vi "Write.vi"(6 "Data":u8[](array[numeric]), 8 "Error In":errorcluster, 9 "Offset":i32 format="%.0x", 10 "Index Group":u32 format="%.0x", 11 "AMS Connection In":T1) -> (0 "Error Out":errorcluster, 1 "Success":bool, 2 "ADS Error":T3 items=["NoError"=0, "InternalError"=1, "NoRTime"=2, "LockedMemoryError"=3, "MailBoxError"=4, "WrongHMsg"=5, "TargetPortNotFound"=6, "TargetMachineNotFound"=7, "UnknownCommandID"=8, "BadTaskID"=9, "NoIO"=10, "UnknownAmsCommand"=11, "Win32Error"=12, "PortNotConnected"=13, "InvalidAmsLength"=14, "InvalidAmsNetID"=15, "AmsSyncAmsError"=22, "AmsSyncNoIndexMap"=23, "InvalidAmsPort"=24, "NoMemory"=25, "TCPSendError"=26, "HostUnreachable"=27, "NoLockedMemory"=1280, "MailboxFull"=1282, "DeviceError"=1792, "DeviceServiceNotSupported"=1793, "DeviceInvalidGroup"=1794, "DeviceInvalidOffset"=1795, "DeviceInvalidAccess"=1796, "DeviceInvalidSize"=1797, "DeviceInvalidData"=1798, "DeviceNotReady"=1799, "DeviceBusy"=1800, "DeviceInvalidContext"=1801, "DeviceNoMemory"=1802, "DeviceInvalidParam"=1803, "DeviceNotFound"=1804, "DeviceSyntaxError"=1805, "DeviceIncompatible"=1806, "DeviceExists"=1807, "DeviceSymbolNotFound"=1808, "DeviceSymbolVersionInvalid"=1809, "DeviceInvalidState"=1810, "DeviceTransModeNotSupported"=1811, "DeviceNotifyHandleInvalid"=1812, "DeviceClientUnknown"=1813, "DeviceNoMoreHandles"=1814, "DeviceInvalidWatchsize"=1815, "DeviceNotInitialized"=1816, "DeviceTimeOut"=1817, "DeviceNoInterface"=1818, "DeviceInvalidInterface"=1819, "DeviceInvalidCLSID"=1820, "DeviceInvalidObjectID"=1821, "ClientError"=1856, "ClientInvalidParameter"=1857, "ClientListEmpty"=1858, "ClientVariableInUse"=1859, "ClientDuplicateInvokeID"=1860, "ClientSyncTimeOut"=1861, "ClientW32OR"=1862, "ClientTimeoutInvalid"=1863, "ClientPortNotOpen"=1864, "ClientNoAmsAddr"=1865, "ClientSyncInternal"=1872, "ClientAddHash"=1873, "ClientRemoveHash"=1874, "ClientNoMoreSymbols"=1875, "ClientSyncResInvalid"=1876, "ClientSyncPortLocked"=1877, "ClientQueueFull"=1878], 3 "AMS Connection Out":T1)   [LabVIEW 2019, in "TwinCAT ADS.lvlib"]
uses:
  <userlib>/PMA/TwinCAT ADS.lvlib
  <userlib>/PMA/Low Level/TypeDefs/AMS Connection.ctl
  <userlib>/PMA/Low Level/TypeDefs/AMS.ctl
  <userlib>/PMA/Low Level/TypeDefs/ADS Error.ctl
  <userlib>/PMA/Low Level/TypeDefs/Command Id.ctl
  <userlib>/PMA/Low Level/TypeDefs/State Flag.ctl
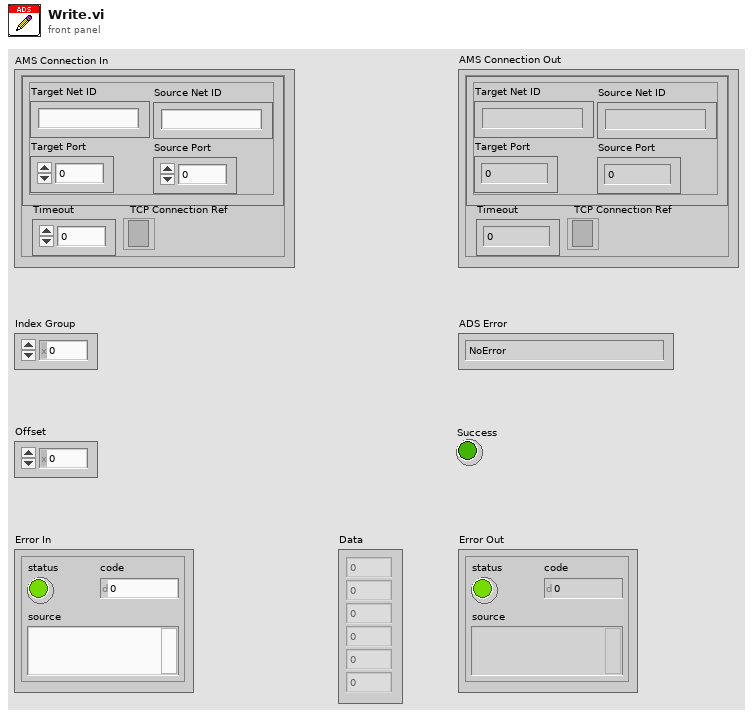
[diagram p1: front panel]
types:
  T1 = typedef "TwinCAT ADS.lvlib/AMS Connection.ctl" = cluster{"AMS":T2, "Timeout":i32, "TCP Connection Ref":refnum<k5>}
  T2 = typedef "TwinCAT ADS.lvlib/AMS.ctl" = cluster{"Target Net ID":string, "Target Port":u16, "Source Net ID":string, "Source Port":u16}
  T3 = typedef "TwinCAT ADS.lvlib/ADS Error.ctl" = i32
  T4 = enum16{"Standard", "Buffered", "CRLF", "Immediate"}
  T5 = typedef "TwinCAT ADS.lvlib/State Flag.ctl" = u16
  T6 = typedef "TwinCAT ADS.lvlib/Command Id.ctl" = enum16{"Invalid", "ADS Read Device Info", "ADS Read", "ADS Write", "ADS Read State", "ADS Write Control", "ADS Add Device Notification", "ADS Delete Device Notification", "ADS Device Notification", "ADS Read Write"}
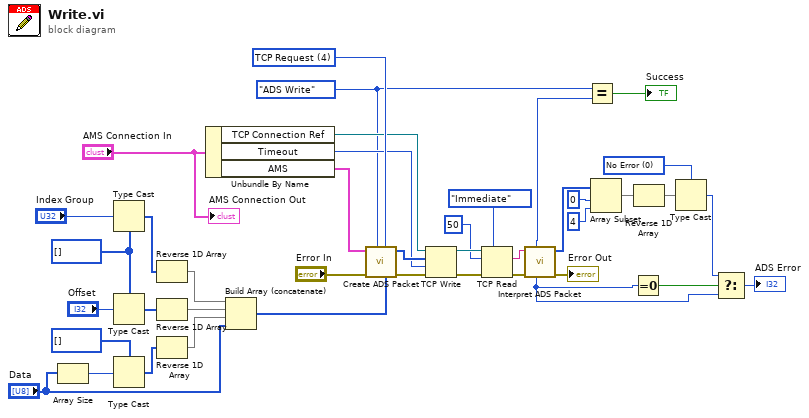
[diagram p0: block diagram]
diagram:
  w22 = T3 0 items=["No Error"] ("Enum")
  w11 = u8[] [] ("bytes to read")
  w41 = T5 4 items=["TCP Request"=4, "TCP Response"=5, "UDP Request"=68, "UDP Respone"=69] ("State Flag")
  w2 = Command_Id."ADS Write" ("Command ID")
  n1 = Array Size(array="Data") -> (size(s)=w9:i32)
  n2 = Type Cast(type=w11, x="Index Group") -> (*(type *) &x=w29:u8[])
  n3 = Type Cast(type=w11, x="Offset") -> (*(type *) &x=w28:u8[])
  n4 = Type Cast(type=u8[] [] ("bytes to read"), x=w9) -> (*(type *) &x=w27:u8[])
  n5 = Reverse 1D Array(array=w29) -> (reversed array=w19:u8[])
  n6 = Reverse 1D Array(array=w28) -> (reversed array=w18:u8[])
  n7 = Reverse 1D Array(array=w27) -> (reversed array=w17:u8[])
  n8 = Unbundle By Name("AMS Connection In") -> ("TCP Connection Ref"=w5:refnum<k5>, "Timeout"=w4:i32, "AMS"=w6:T2)
  n9 = Build Array (concatenate)(w19, w18, w17, "Data") -> (w26:u8[])
  n10 = call <userlib>:"Create ADS Packet.vi"("Data"=w26, "State Flag"=w41, "Command ID"=w2, "Error In"="Error In", "AMS"=w6) -> ("Error Out"=w38:errorcluster, "ADS Packet"=w40:u8[])  [unwired: 5 in]
  n11 = TCP Write(connection ID=w5, data in=w40, error in (no error)=w38, 9:w4) -> (connection ID out=w39:refnum<k5>, error out=w37:errorcluster)  [unwired: 1 out]
  n12 = TCP Read(connection ID=w39, bytes to read=u32 50, error in (no error)=w37, 7:T4."Immediate" ("mode (standard)")) -> (data out=w33:string, error out=w34:errorcluster)  [unwired: 1 in, 1 out]
  n13 = call <userlib>:"Interpret ADS Packet.vi"("Error In"=w34, "ADS Packet"=w33) -> ("Error Out"=→"Error Out":errorcluster, "Data"=w21:u8[], "ADS Error"=w13:T3, "Command ID"=w3:T6)  [unwired: 3 in, 3 out]
  n14 = Equal?(x=w2, y=w3) -> (x = y?=→"Success":bool)
  n15 = Array Subset(array=w21, index=0, length=4) -> (w23:u8[])
  n16 = Equal To 0?(x=w13) -> (x = 0?=w15:bool)
  n17 = Reverse 1D Array(array=w23) -> (reversed array=w16:u8[])
  n18 = Type Cast(type=w22, x=w16) -> (*(type *) &x=w14:T3)
  n19 = Select(t=w14, s=w15, f=w13) -> (s? t:f=→"ADS Error":T3)
  "AMS Connection Out" <- "AMS Connection In"
